vi "removeItem.vi"(8 "error in (no error)":errorcluster, 10 "Key":string, 11 "Bucket in":refnum<class "Bucket.lvclass">) -> (0 "error out":errorcluster, 3 "Bucket out":refnum<class "Bucket.lvclass">)   [LabVIEW 2017, in "Bucket.lvclass"]
uses:
  <userlib>/836-Library/Data_Structures/HashMap/Support/Bucket/Bucket.lvclass
  <userlib>/836-Library/Data_Structures/HashMap/Support/Bucket/Bucket.lvclass/Bucket.ctl
  <userlib>/836-Library/Data_Structures/HashMap/Support/Bucket/Types/KeyValuePair.ctl
  <vilib>/Utility/error.llb/Error Cluster From Error Code.vi
  <vilib>/ErrorRing/Error Ring.xnode
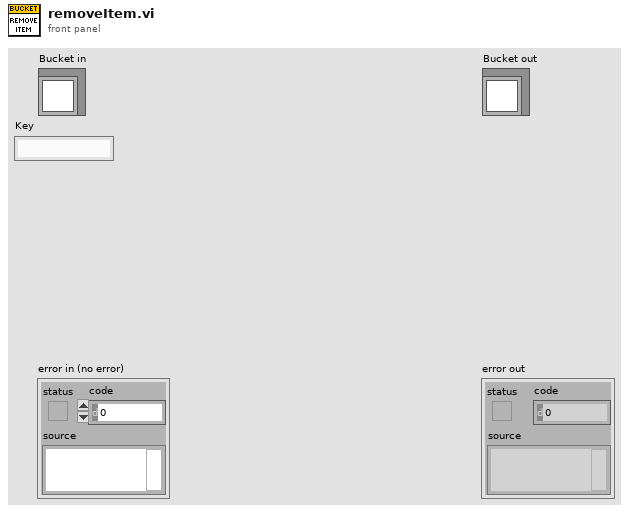
[diagram p1: front panel]
types:
  T1 = typedef "KeyValuePair.ctl" = cluster{"Key":string, "Value":variant}
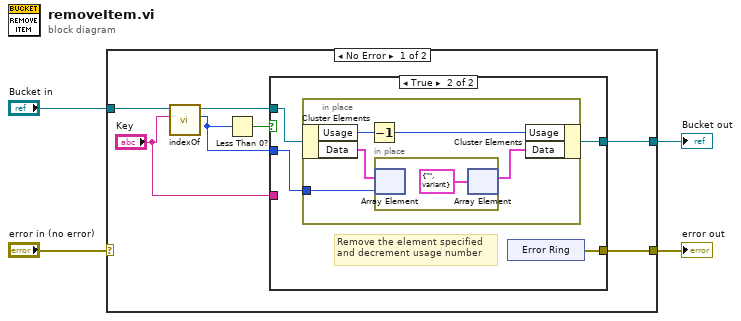
[diagram p0: block diagram]
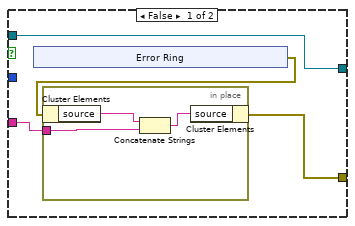
[diagram p2: hidden frame]
diagram:
  n1 = case shown="No Error" "error in (no error)" {
    selector: "error in (no error)" -> [_ w36]
    tunnel: [w5 w36] -> w3
    tunnel: [w7 w35] -> w1
    tunnel: "Bucket in" -> [w11 w35]
    frame No Error {
      n2 = call <userlib>:"indexOf.vi"("Key"="Key", "Bucket in"=w11) -> ("Index"=w8:i32, "Bucket out"=w10:refnum<class "Bucket.lvclass">)  [unwired: 7 in, 1 out]
      n3 = Less Than 0?(x=w8) -> (x < 0?=w9:bool)
      n4 = case shown="True" w9 {
        tunnel: w10 -> [w15 w27]
        tunnel: w8 -> [_ w26]
        tunnel: [w15 w25] -> w7
        tunnel: "Key" -> [w13 _]
        tunnel: [w12 w24] -> w5
        frame False {
          n5 = xnode "Error Ring"() -> ("error out"=w14:errorcluster)
          n6 = in-place {
            in-place-border: w13 -> [w16]
            n7 = in-place-cluster #1(w14) -> ("source"=w17:string)
            n8 = Concatenate Strings(w17, w16) -> (w18:string)
            n9 = in-place-cluster #1("source"=w18) -> (w12:errorcluster)
          }
        }
        frame True {
          # "Remove the element specified\nand decrement usage number"
          n10 = in-place {
            in-place-border: w26 -> [w30]
            n11 = in-place-cluster #2(w27) -> ("Usage"=w32:u32, "Data"=w31:T1[])
            n12 = Decrement(x=w32) -> (x-1=w33:u32)
            n13 = in-place {
              n14 = in-place-array #3(w31, w30) -> ()  [unwired: 1 out]
              n15 = in-place-array #3(T1 {"Key"="", "Value"=variant} ("element")) -> (w29:T1[])  [unwired: 1 out]
            }
            n16 = in-place-cluster #2("Usage"=w33, "Data"=w29) -> (w25:refnum<class "Bucket.lvclass">)
          }
          n17 = xnode "Error Ring"() -> ("error out"=w24:errorcluster)
        }
      }
    }
    frame Error {
    }
  }
  "error out" <- w3
  "Bucket out" <- w1
